vi "Name to Queue.vi"(0 "Queue Name in":string) -> (5 "Found?":bool, 6 "Queue out":refnum<queue>)   [LabVIEW 2018, in "Queue.lvlib"]
uses:
  Queue.lvlib
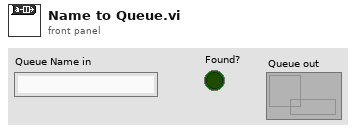
[diagram p1: front panel]
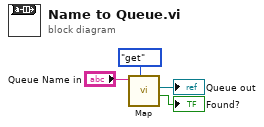
[diagram p0: block diagram]
diagram:
  n1 = call "Map.vi"("Action"=enum8{"noop", "get", "set", "pop"}."get", "Queue Name"="Queue Name in") -> ("Found?"=→"Found?":bool, "Queue out"=→"Queue out":refnum<queue>)  [unwired: 8 in]
